vi "test_pathProject.vi"(8 "error in (no error)":errorcluster) -> (0 "error out":errorcluster)   [LabVIEW 2013]
uses:
  Run Test (Scalar Path).vi
  Caraya.lvlib
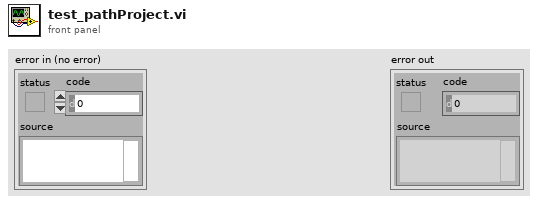
[diagram p1: front panel]
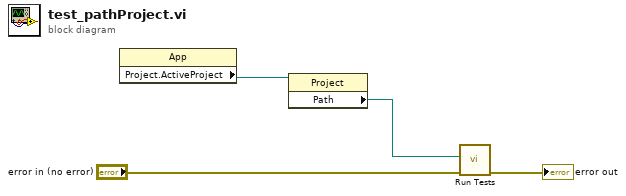
[diagram p0: block diagram]
diagram:
  n1 = property class="App"() -> ("Project.ActiveProject"=w2:refnum<vi>)  [unwired: 2 in, 2 out]
  n2 = property class="Project"(reference=w2) -> ("Path"=w1:path)  [unwired: 1 in, 2 out]
  n3 = call-poly "Run Tests.vi"("error in"="error in (no error)", "Test Path"=w1) -> ("error out"=→"error out":errorcluster)  [unwired: 9 in]
